vi "Adjust List Column.vi"(8 "error in (no error)":errorcluster caption="错误输入（无错误）", 10 "Column":i32, 11 "MCListBox in":refnum<vi>) -> (0 "error out":errorcluster caption="错误输出", 3 "MCListBox out":refnum<vi>)   [LabVIEW 2013]
uses:
  <vilib>/Utility/miscctls.llb/LVRowAndColumnTypeDef.ctl
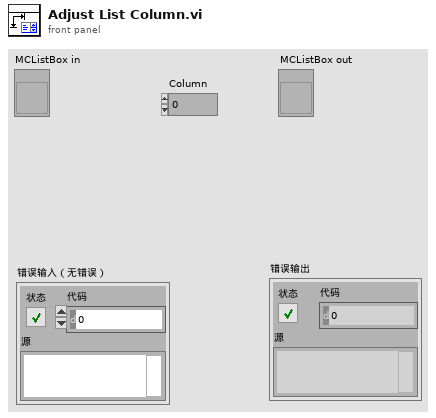
[diagram p1: front panel]
types:
  T1 = typedef "LVRowAndColumnTypeDef.ctl" = cluster{"Row":i32, "Column":i32}
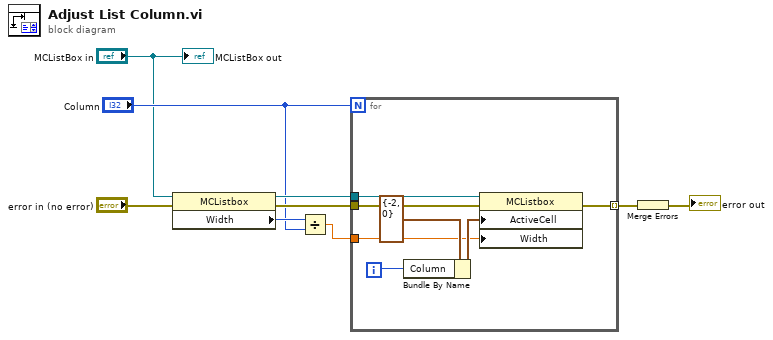
[diagram p0: block diagram]
diagram:
  n1 = property class="MCListbox"(reference="MCListBox in", error in="error in (no error)") -> (reference out=w9:refnum<vi>, error out=w8:errorcluster, "Width"=w7:u32)
  n2 = Divide(x=w7, y="Column") -> (x/y=w5:dbl)
  n3 = for {
    N: "Column" -> [_]
    tunnel: w9 -> [w16]
    tunnel: w8 -> [w15]
    tunnel: w5 -> [w11]
    tunnel: [w10] -> w4 mode=indexing
    i -> [w12]
    n4 = Bundle By Name(cluster=T1 {"Row"=-2, "Column"=0} ("活动单元格:活动单元格"), "Column"=w12) -> (w13:T1)
    n5 = property class="MCListbox"(reference=w16, error in=w15, "ActiveCell"=w13, "Width"=w11) -> (error out=w10:errorcluster)  [unwired: 1 out]
  }
  n6 = Merge Errors(w4) -> (→"error out":errorcluster)
  "MCListBox out" <- "MCListBox in"
